vi "test Disabled Device can be Deployed.vi"(8 "error in (no error)":errorcluster, 11 "TestCase in":refnum<class "Disabled Custom Device.lvclass">) -> (0 "error out":errorcluster, 3 "TestCase out":refnum<class "Disabled Custom Device.lvclass">)   [LabVIEW 2020, in "Disabled Custom Device.lvclass"]
uses:
  Disabled Custom Device.lvclass
  Disabled Custom Device.lvclass/Disabled Custom Device.ctl
  <vilib>/addons/_JKI Toolkits/VI Tester/TestCase.llb/TestCase.lvclass
  C:/dev/git/niveristand-custom-device-testing-tools/VeriStandTestCase/VeriStandTestCase.lvclass
  C:/Program Files (x86)/National Instruments/LabVIEW 2020/vi.lib/addons/_JKI Toolkits/VI Tester/TestCase.llb/TestCase.lvclass
  C:/dev/git/niveristand-ballard-milStd1553-custom-device/Source/Custom Device Support/Tests/System/Disabled Custom Device/Disabled Custom Device.lvclass
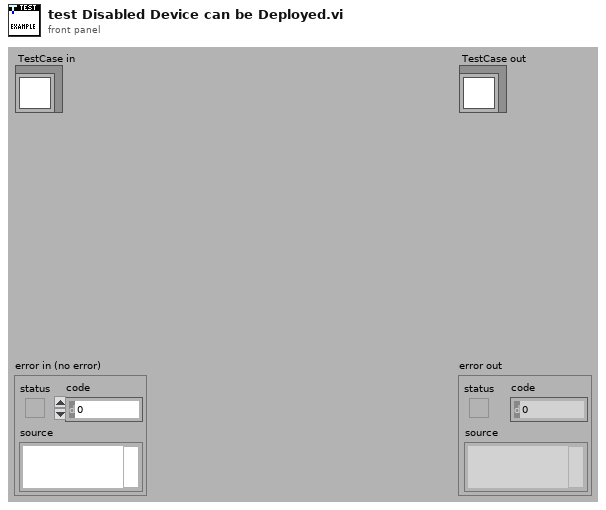
[diagram p1: front panel]
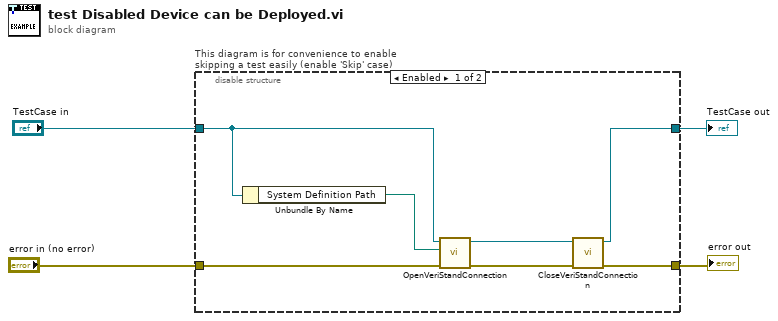
[diagram p0: block diagram]
diagram:
  n1 = disable-structure "This diagram is for convenience to enable skipping a test easily (enable 'Skip' case)" shown="Enabled" {
    disable-tunnel: "TestCase in" -> [w8 w15]
    disable-tunnel: [w5 w13] -> w1
    disable-tunnel: [w6 w14] -> w3
    disable-tunnel: "error in (no error)" -> [w11 w12]
    frame Enabled {
      n2 = Unbundle By Name(w8) -> ("System Definition Path"=w9:path)
      n3 = call-dynamic "OpenVeriStandConnection.vi"("error in (no error)"=w11, "System Definition File"=w9, "VeriStand Test Case in"=w8) -> ("error out"=w10:errorcluster, "VeriStand Test Case out"=w7:refnum<class "Disabled Custom Device.lvclass">)  [unwired: 6 in, 1 out]
      n4 = call-dynamic "CloseVeriStandConnection.vi"("error in (no error)"=w10, "VeriStand Test Case in"=w7) -> ("error out"=w6:errorcluster, "VeriStand Test Case out"=w5:refnum<class "Disabled Custom Device.lvclass">)  [unwired: 8 in]
    }
    frame Disabled {
      # "skip test result while test is under development"
      n5 = call <vilib>:"skip.vi"("error in (no error)"=w12, "TestCase in"=w15) -> ("error out"=w14:errorcluster, "TestCase out"=w13:refnum<class "Disabled Custom Device.lvclass">)  [unwired: 8 in]
    }
  }
  "error out" <- w3
  "TestCase out" <- w1
